vi "light_task.vi"() -> ()   [LabVIEW 2023]
uses:
  <vilib>/DAQmx/read.llb/DAQmx Read (Analog DBL 1Chan 1Samp).vi
  <vilib>/DAQmx/write.llb/DAQmx Write (Digital 1D Bool NChan 1Samp 1Line).vi
  <vilib>/DAQmx/miscellaneous.llb/DAQmx Fill In Error Info.vi
panel:
  out "data":bool[](array[boolean])
  out "millisecond timer value":u32
  in  "stop":bool
  out "Waveform Chart":dbl(graph)
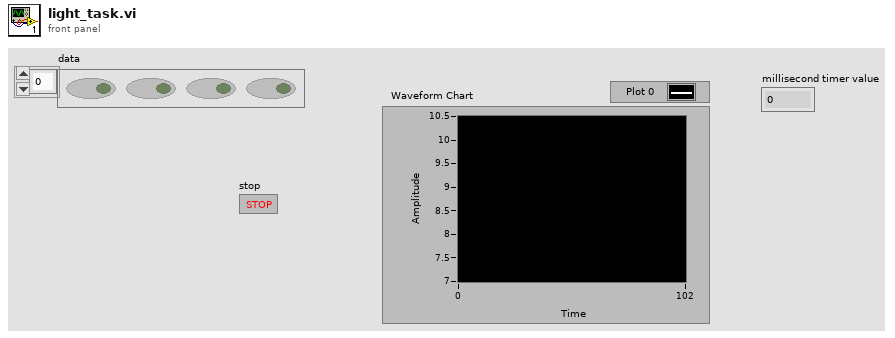
[diagram p1: front panel]
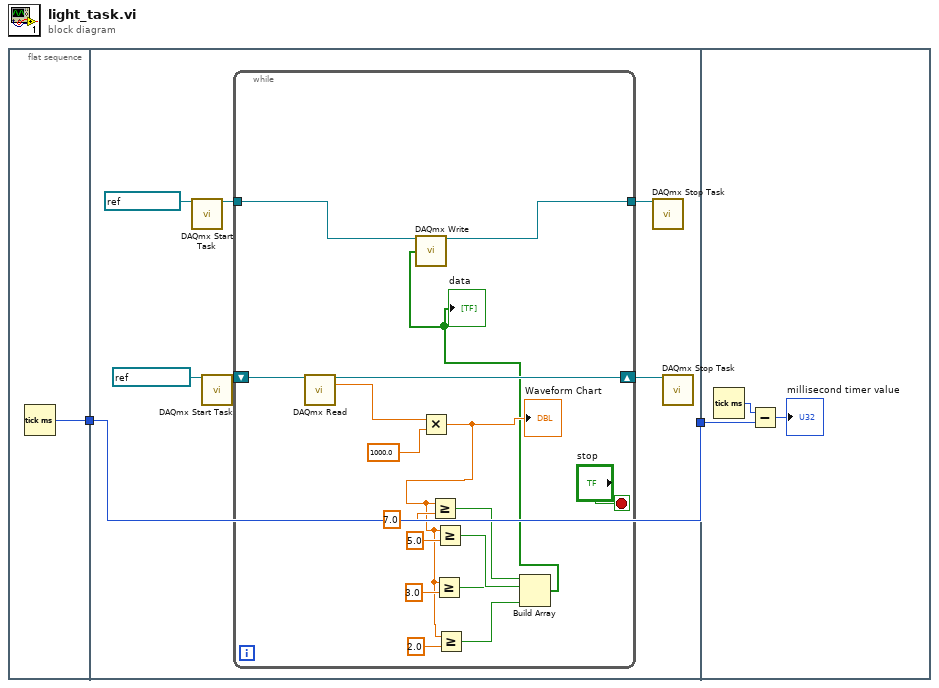
[diagram p0: block diagram]
diagram:
  n1 = flat-sequence {
    tunnel: [w3] -> w1
    tunnel: [w7] -> w2
    tunnel: w1 -> [w7]
    tunnel: w2 -> [w28]
    frame #0 {
      n2 = Tick Count (ms)() -> (millisecond timer value=w3:u32)
    }
    frame #1 {
      n3 = call <vilib>:"DAQmx Start Task.vi"("task/channels in"=refnum<k21> "LED_Task") -> ("task out"=w5:refnum<k21>)  [unwired: 13 in, 1 out]
      n4 = call <vilib>:"DAQmx Start Task.vi"("task/channels in"=refnum<k21> "LightTask") -> ("task out"=w10:refnum<k21>)  [unwired: 13 in, 1 out]
      n5 = while {
        shift-right: [w26] -> w9
        shift-left: w10 -> [w27]
        tunnel: w5 -> [w22]
        tunnel: [w21] -> w4
        stop <- "stop" stop-if-true
        n6 = call-poly <vilib>:"DAQmx Read.vi"("task/channels in"=w27) -> ("task out"=w26:refnum<k21>, "data"=w24:dbl)  [unwired: 12 in, 1 out]
        n7 = Multiply(x=w24, y=1000.0) -> (x*y=w17:dbl)
        "Waveform Chart" <- w17
        n8 = Greater Or Equal?(x=w17, y=7.0) -> (x >= y?=w15:bool)
        n9 = Greater Or Equal?(x=w17, y=3.0) -> (x >= y?=w13:bool)
        n10 = Greater Or Equal?(x=w17, y=5.0) -> (x >= y?=w14:bool)
        n11 = Greater Or Equal?(x=w17, y=2.0) -> (x >= y?=w12:bool)
        n12 = Build Array(w15, w14, w13, w12) -> (w11:bool[])
        "data" <- w11
        n13 = call-poly <vilib>:"DAQmx Write.vi"("task/channels in"=w22, "data"=w11) -> ("task out"=w21:refnum<k21>)  [unwired: 11 in, 2 out]
      }
      n14 = call <vilib>:"DAQmx Stop Task.vi"("task/channels in"=w4) -> ()  [unwired: 13 in, 2 out]
      n15 = call <vilib>:"DAQmx Stop Task.vi"("task/channels in"=w9) -> ()  [unwired: 13 in, 2 out]
    }
    frame #2 {
      n16 = Tick Count (ms)() -> (millisecond timer value=w29:u32)
      n17 = Subtract(x=w29, y=w28) -> (x-y=→"millisecond timer value":u32)
    }
  }
